vi "v1.92. vi.vi"() -> ()   [LabVIEW 2018]
uses:
  <vilib>/Analysis/baseanly.llb/Mean (DBL).vi
  <vilib>/DAQmx/read.llb/DAQmx Read (Analog 1D DBL NChan 1Samp).vi
  <extravilib>/ChannelInstances/High Speed Stream-a[.](dbl)/_Read For Replicate.vi
  <vilib>/DAQmx/create/channels.llb/DAQmx Create Channel (AI-Voltage-Basic).vi
  <vilib>/DAQmx/configure/timing.llb/DAQmx Timing (Sample Clock).vi
  <extravilib>/ChannelInstances/High Speed Stream-a[.](dbl)/Instantiate.vi
  <extravilib>/ChannelInstances/High Speed Stream-a[.](dbl)/)Channel.vi
  <extravilib>/ChannelInstances/High Speed Stream-a[.](dbl)/Abort Signal/Init Signal.vi
  <vilib>/DAQmx/miscellaneous.llb/DAQmx Fill In Error Info.vi
  <extravilib>/ChannelInstances/High Speed Stream-a[.](dbl).lvlib
  <vilib>/Analysis/NI_AALBase.lvlib
panel:
  out "Mixed Signal Graph":T1(graph)
  out "Global Stop Indicator":bool=TRUE
  in  "Global Stop":bool
  in  "Avg Of?":dbl
  in  "Record?":bool
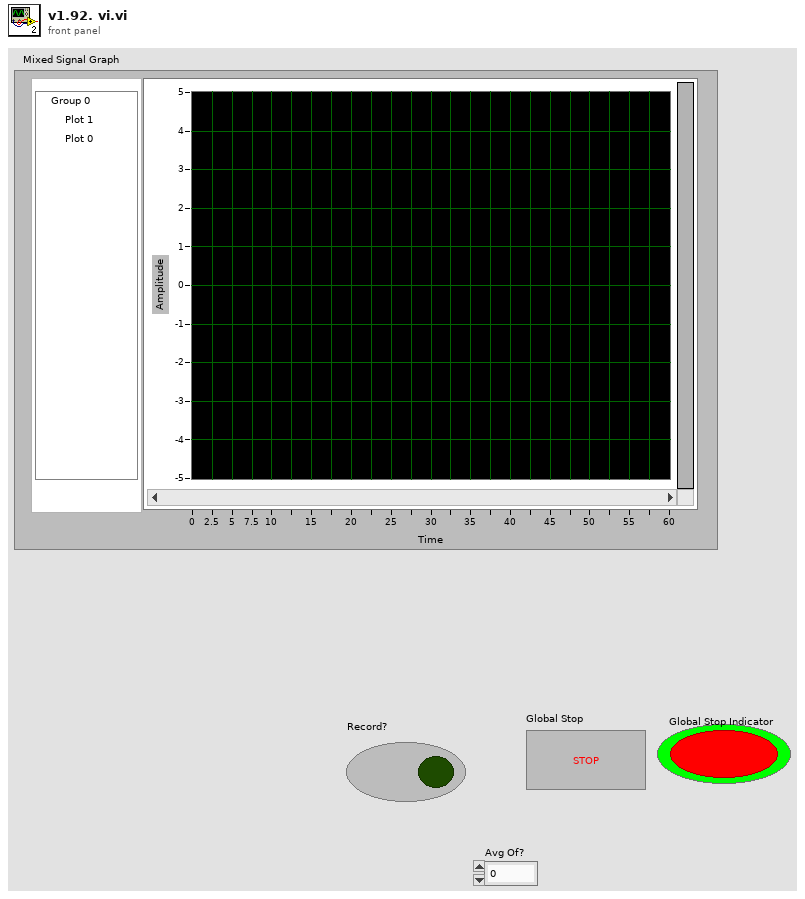
[diagram p1: front panel]
types:
  T1 = cluster{"Time":dbl, "Signal 1":dbl, "Signal 2":dbl}[]
  T2 = typedef "High Speed Stream-a[.](dbl).lvlib/)Channel.ctl" = refnum<queue>
  T3 = cluster{"Time":dbl, "Signal 1":dbl, "Signal 2":dbl}
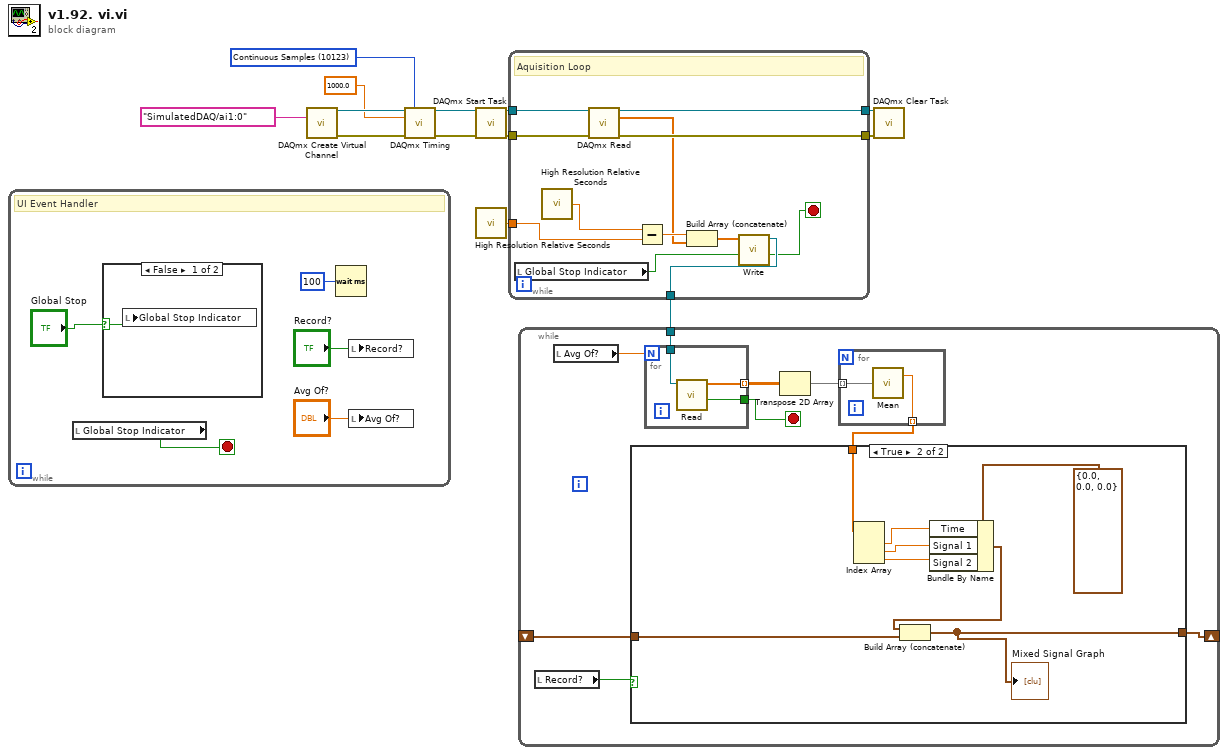
[diagram p0: block diagram]
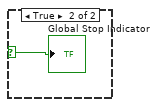
[diagram p3: hidden frame]
diagram:
  w9 = 10123 items=["Finite Samples"=10178, "Continuous Samples"=10123, "Hardware Timed Single Point"=12522] ("sample mode")
  n1 = while {
    stop <- w14 stop-if-true
    # "UI Event Handler"
    n2 = local read "Global Stop Indicator"() -> (w14:bool)
    n3 = case shown="False" "Global Stop" {
      selector: "Global Stop" -> [w19 w20]
      frame False {
        n4 = local write "Global Stop Indicator"(w19) -> ()
      }
      frame True {
        "Global Stop Indicator" <- w20
      }
    }
    n5 = Wait (ms)(milliseconds to wait=u32 100) -> ()  [unwired: 1 out]
    n6 = local write "Record?"("Record?") -> ()
    n7 = local write "Avg Of?"("Avg Of?") -> ()
  }
  n8 = call-poly <vilib>:"DAQmx Create Virtual Channel.vi"("physical channels"=tag "SimulatedDAQ/ai1:0") -> ("task out"=w10:refnum<k21>, "error out"=w11:errorcluster)  [unwired: 13 in]
  n9 = call-poly <vilib>:"DAQmx Timing.vi"("task/channels in"=w10, "sample mode"=w9, "rate"=1000.0, "error in"=w11) -> ("task out"=w12:refnum<k21>, "error out"=w13:errorcluster)  [unwired: 10 in]
  n10 = call <vilib>:"DAQmx Start Task.vi"("task/channels in"=w12, "error in"=w13) -> ("task out"=w3:refnum<k21>, "error out"=w4:errorcluster)  [unwired: 12 in]
  n11 = call <vilib>:"High Resolution Relative Seconds.vi"() -> ("relative seconds"=w2:dbl)
  n12 = while {
    tunnel: w3 -> [w29]
    tunnel: w4 -> [w32]
    tunnel: [w31] -> w7
    tunnel: [w30] -> w6
    tunnel: w2 -> [w27]
    tunnel: [w25] -> w1
    stop <- w23 stop-if-true
    # "Aquisition Loop"
    n13 = local read "Global Stop Indicator"() -> (w24:bool)
    n14 = call <vilib>:"High Resolution Relative Seconds.vi"() -> ("relative seconds"=w28:dbl)
    n15 = call-poly <vilib>:"DAQmx Read.vi"("task/channels in"=w29, "error in"=w32) -> ("task out"=w31:refnum<k21>, "data"=w22:dbl[], "error out"=w30:errorcluster)  [unwired: 11 in]
    n16 = Subtract(x=w28, y=w27) -> (x-y=w26:dbl)
    n17 = Build Array (concatenate)(w26, w22) -> (w21:dbl[])
    n18 = call <extravilib>:"Write.vi"("last element? (F)"=w24, "element"=w21) -> ("done?"=w23:bool, "channel"=w25:T2)  [unwired: 7 in, 1 out]
  }
  n19 = while {
    tunnel: w1 -> [w40]
    shift-right: [w34] -> _
    shift-left: _ -> [w35]
    stop <- w37 stop-if-true
    n20 = local read "Record?"() -> (w33:bool)
    n21 = local read "Avg Of?"() -> (w41:dbl)
    n22 = for {
      N: w41 -> [_]
      tunnel: w40 -> [w55]
      tunnel: [w54] -> w39 mode=indexing
      tunnel: [w53] -> w37
      n23 = call <extravilib>:"Read.vi"("channel"=w55) -> ("done?"=w53:bool, "element"=w54:dbl[])  [unwired: 6 in, 3 out]
    }
    n24 = Transpose 2D Array(2D array=w39) -> (transposed array=w38:dbl[][])
    n25 = for {
      tunnel: w38 -> [w52] mode=indexing
      tunnel: [w51] -> w36 mode=indexing
      n26 = call-poly <vilib>:"Mean.vi"("X"=w52) -> ("mean"=w51:dbl)  [unwired: 1 out]
    }
    n27 = case shown="True" w33 {
      tunnel: w36 -> [_ w50]
      tunnel: w35 -> [w42 w46]
      tunnel: [w42 w43] -> w34
      frame False {
      }
      frame True {
        n28 = Index Array(array=w50) -> (element #1=w49:dbl, element #2=w48:dbl, element #3=w47:dbl)  [unwired: 3 in]
        n29 = Bundle By Name(cluster=T3 {"Time"=0.0, "Signal 1"=0.0, "Signal 2"=0.0} ("input cluster"), "Time"=w49, "Signal 1"=w48, "Signal 2"=w47) -> (w44:T3)
        n30 = Build Array (concatenate)(w44, w46) -> (w43:T1)
        "Mixed Signal Graph" <- w43
      }
    }
  }
  n31 = call <vilib>:"DAQmx Clear Task.vi"("task in"=w7, "error in"=w6) -> ()  [unwired: 13 in, 1 out]
